vi "LinearAndAngularProfileGenerator.vi"(0 "Radius":dbl=60.0, 1 "MaxVelAngular":dbl=inf, 2 "MaxAccelAngular":dbl=inf, 5 "Theta":dbl=90.0, 7 "InitialVelocity":dbl, 9 "FinalVelocity":dbl, 11 "dt":u32=20, 12 "MaxVelocity":dbl=100.0, 13 "MaxAccel":dbl=75.0) -> (4 "Pos":dbl[](array[numeric]), 6 "Vel":dbl[](array[numeric]), 8 "AnglePos":dbl[](array[numeric]), 10 "AngularVel":dbl[](array[numeric]), 15 "dt":u32=20)   [LabVIEW 2016]
panel:
  out "Angle":dbl[][](graph)
  out "Linear":dbl[][](graph)
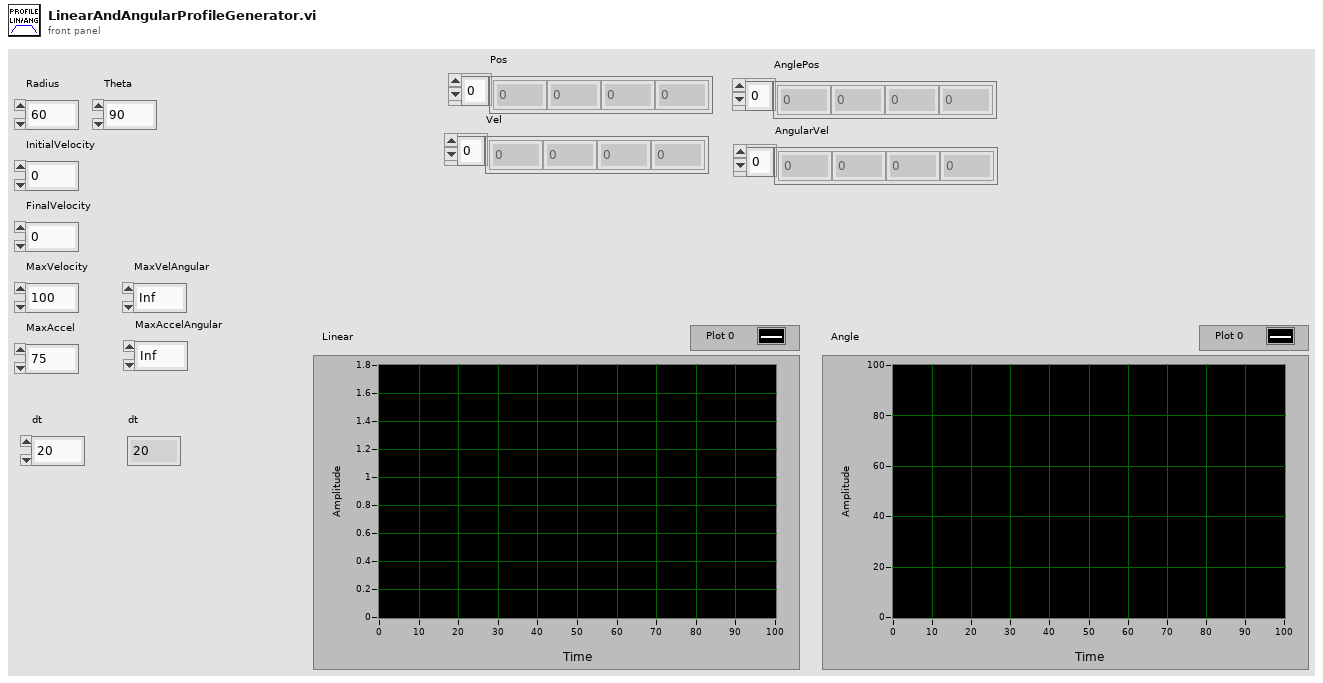
[diagram p1: front panel]
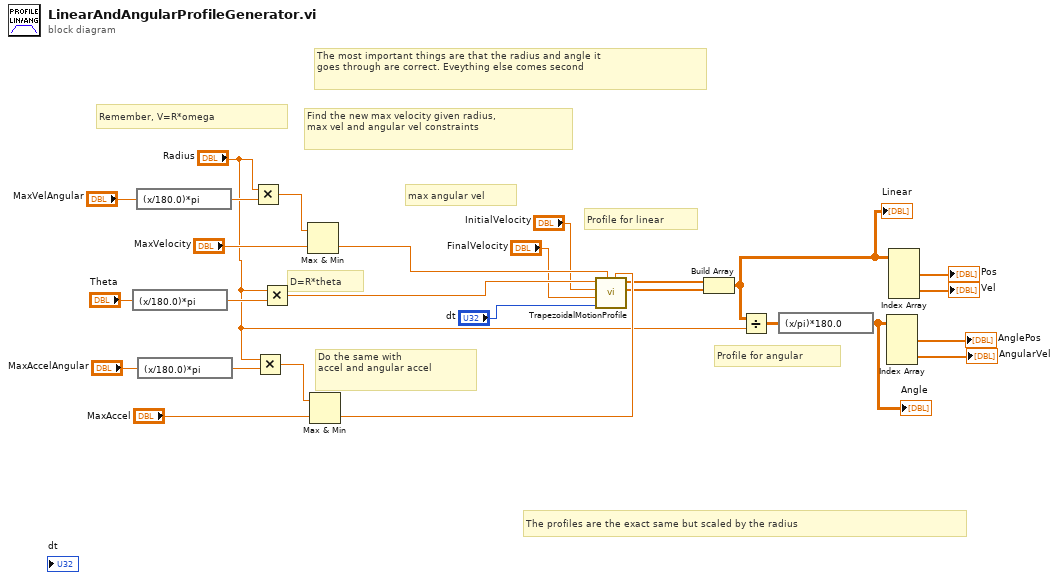
[diagram p0: block diagram]
diagram:
  # "The profiles are the exact same but scaled by the radius"
  # "D=R*theta"
  # "Profile for angular"
  # "Profile for linear"
  # "Do the same with\naccel and angular accel"
  # "max angular vel"
  # "Find the new max velocity given radius, \nmax vel and angular vel constraints"
  # "The most important things are that the radius and angle it \ngoes through are correct. Eveything else comes second"
  # "Remember, V=R*omega"
  n1 = expression code="(x/180.0)*pi" ("degrees to radians")("Theta") -> (w11:dbl)
  n2 = expression code="(x/180.0)*pi" ("degrees to radians")("MaxVelAngular") -> (w14:dbl)
  n3 = expression code="(x/180.0)*pi" ("degrees to radians")("MaxAccelAngular") -> (w15:dbl)
  n4 = Multiply(x="Radius", y=w14) -> (x*y=w26:dbl)
  n5 = Multiply(x="Radius", y=w15) -> (x*y=w24:dbl)
  n6 = Multiply(x="Radius", y=w11) -> (x*y=w22:dbl)
  n7 = Max & Min(x=w26, y="MaxVelocity") -> (min(x,y)=w21:dbl)  [unwired: 1 out]
  n8 = Max & Min(x=w24, y="MaxAccel") -> (min(x,y)=w20:dbl)  [unwired: 1 out]
  n9 = call "TrapezoidalMotionProfile.vi"("MaxAccel"=w20, "MaxVelocity"=w21, "dt"="dt", "FinalVelocity"="FinalVelocity", "InitialVelocity"="InitialVelocity", "Distance"=w22) -> ("Vel"=w17:dbl[], "Pos"=w18:dbl[])  [unwired: 2 in, 2 out]
  n10 = Build Array(w18, w17) -> (w5:dbl[][])
  "Linear" <- w5
  n11 = Divide(x=w5, y="Radius") -> (x/y=w9:dbl[][])
  n12 = expression code="(x/pi)*180.0" ("radians to degrees")(w9) -> (w6:dbl[][])
  "Angle" <- w6
  n13 = Index Array(array=w6) -> (element #1=→"AnglePos":dbl[], element #2=→"AngularVel":dbl[])  [unwired: 4 in]
  n14 = Index Array(array=w5) -> (element #1=→"Pos":dbl[], element #2=→"Vel":dbl[])  [unwired: 4 in]
